vi "GetRandomString.vi"(8 "error in (no error)":errorcluster, 11 "Generator in":refnum<class "Generator.lvclass">) -> (0 "error out":errorcluster, 3 "Generator out":refnum<class "Generator.lvclass">)   [LabVIEW 2021, in "Generator.lvlib" / "Generator.lvclass"]
uses:
  Generator.lvclass
  Generator.lvclass/Generator.ctl
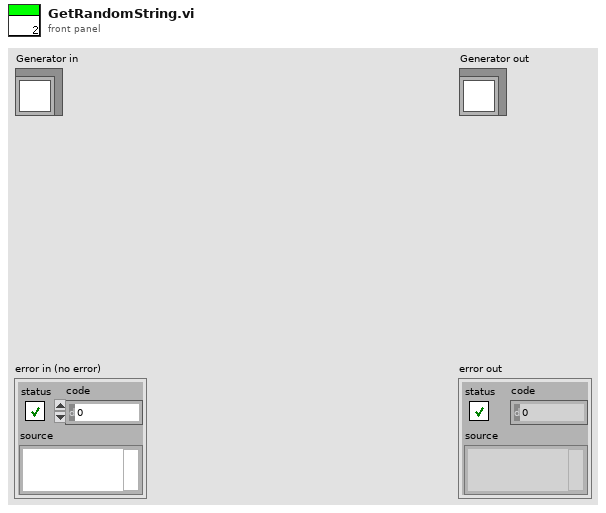
[diagram p1: front panel]
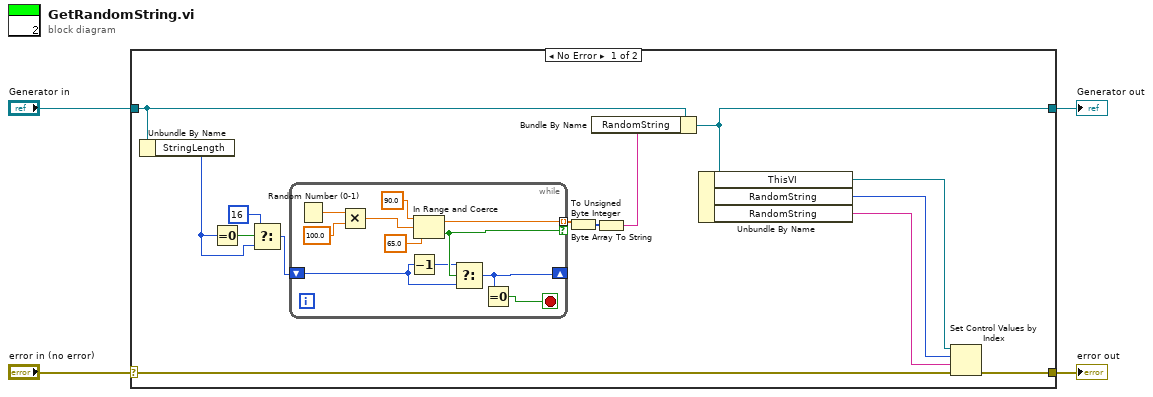
[diagram p0: block diagram]
diagram:
  n1 = case shown="No Error" "error in (no error)" {
    selector: "error in (no error)" -> [w18 w31]
    tunnel: [w9 w31] -> w3
    tunnel: [w8 w30] -> w1
    tunnel: "Generator in" -> [w14 w30]
    frame No Error {
      n2 = Unbundle By Name(w14) -> ("StringLength"=w12:i32)
      n3 = Equal To 0?(x=w12) -> (x = 0?=w13:bool)
      n4 = Select(t=16, s=w13, f=w12) -> (s? t:f=w10:i32)
      n5 = while {
        tunnel: [w24] -> w17 mode=indexing if=w23
        shift-right: [w20] -> _
        shift-left: w10 -> [w21]
        stop <- w19 stop-if-true
        n6 = Random Number (0-1)() -> (number: 0 to 1=w29:dbl)
        n7 = Multiply(x=w29, y=100.0) -> (x*y=w28:dbl)
        n8 = Decrement(x=w21) -> (x-1=w22:i32)
        n9 = In Range and Coerce(upper limit=90.0, x=w28, lower limit=65.0) -> (coerced(x)=w24:dbl, In Range?=w23:bool)
        n10 = Select(t=w22, s=w23, f=w21) -> (s? t:f=w20:i32)
        n11 = Equal To 0?(x=w20) -> (x = 0?=w19:bool)
      }
      n12 = To Unsigned Byte Integer(number=w17) -> (unsigned 8bit integer=w16:u8[])
      n13 = Byte Array To String(unsigned byte array=w16) -> (string=w15:string)
      n14 = Bundle By Name(cluster=w14, "RandomString"=w15) -> (w8:refnum<class "Generator.lvclass">)
      n15 = Unbundle By Name(w8) -> ("ThisVI"=w7:refnum<vi>, "RandomString"=w6:i32, "RandomString"=w5:string)
      n16 = Set Control Values by Index(0:w7, 1:w6, 2:w5, 3:w18) -> (11:w9:errorcluster)
    }
    frame Error {
    }
  }
  "error out" <- w3
  "Generator out" <- w1
